vi "ModeToHideList.vi"(11 "Value":T2) -> (3 "mode":T1)   [LabVIEW 2017, in "UI_TimeSelector.xctl"]
uses:
  UI_TimeSelector.xctl
  Interface/DEF-Mode.ctl
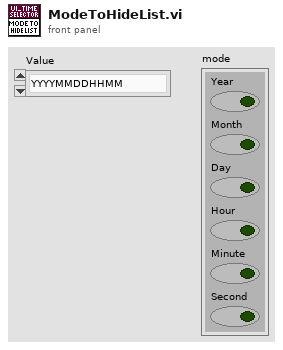
[diagram p1: front panel]
types:
  T1 = cluster{"Year":bool, "Month":bool, "Day":bool, "Hour":bool, "Minute":bool, "Second":bool}
  T2 = typedef "UI_TimeSelector.xctl/DEF-Mode.ctl" = enum16{"YYYYMMDDHHMM", "YYYYMMDDHHMMSS", "YYYY", "YYYYMM", "YYYYMMDD", "HHMM", "HHMMSS"}
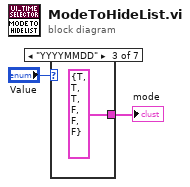
[diagram p0: block diagram]
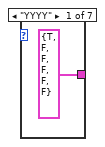
[diagram p2: hidden frame]
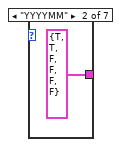
[diagram p3: hidden frame]
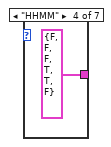
[diagram p4: hidden frame]
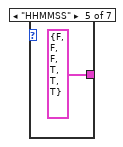
[diagram p5: hidden frame]
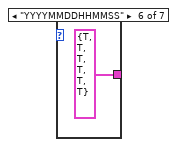
[diagram p6: hidden frame]
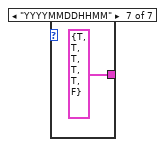
[diagram p7: hidden frame]
diagram:
  n1 = case shown="\"YYYYMMDD\"" "Value" {
    tunnel: [T1 {"Year"=TRUE, "Month"=FALSE, "Day"=FALSE, "Hour"=FALSE, "Minute"=FALSE, "Second"=FALSE} ("mode") T1 {"Year"=TRUE, "Month"=TRUE, "Day"=FALSE, "Hour"=FALSE, "Minute"=FALSE, "Second"=FALSE} ("mode") T1 {"Year"=TRUE, "Month"=TRUE, "Day"=TRUE, "Hour"=FALSE, "Minute"=FALSE, "Second"=FALSE} ("mode") T1 {"Year"=FALSE, "Month"=FALSE, "Day"=FALSE, "Hour"=TRUE, "Minute"=TRUE, "Second"=FALSE} ("mode") T1 {"Year"=FALSE, "Month"=FALSE, "Day"=FALSE, "Hour"=TRUE, "Minute"=TRUE, "Second"=TRUE} ("mode") T1 {"Year"=TRUE, "Month"=TRUE, "Day"=TRUE, "Hour"=TRUE, "Minute"=TRUE, "Second"=TRUE} ("mode") T1 {"Year"=TRUE, "Month"=TRUE, "Day"=TRUE, "Hour"=TRUE, "Minute"=TRUE, "Second"=FALSE} ("mode")] -> w2
    frame "YYYY" {
    }
    frame "YYYYMM" {
    }
    frame "YYYYMMDD" {
    }
    frame "HHMM" {
    }
    frame "HHMMSS" {
    }
    frame "YYYYMMDDHHMMSS" {
    }
    frame "YYYYMMDDHHMM" {
    }
  }
  "mode" <- w2
